vi "Auto-Generate-Docs.vi"(5 "Files Generated by Build":path[](array[path]), 6 "Top Level/Always Included VIs":path[](array[path]), 7 "Destination Path":path, 8 "error in (no error)":errorcluster, 9 "Target Name":string, 10 "Build Specification Name":string, 11 "Project Path":path) -> (0 "error out":errorcluster)   [LabVIEW 2019]
uses:
  <vilib>/printing/EasyPrintingControls.llb/custom_contents_options.ctl
  <vilib>/printing/EasyPrintingControls.llb/list_which_controls.ctl
  <vilib>/AppBuilder/AB_API_Simple/NI_App_Builder_API.lvlib
  <vilib>/AppBuilder/AB_API_Simple/Get Build Specification Version (path).vi
  <vilib>/Utility/NIReport.llb/NI_ReportGenerationCore.lvlib
panel:
  in  "custom contents options":T1={"include VI connector and icon"=TRUE, "include VI description"=TRUE, "include front panel"=FALSE, "surround front panel with border"=FALSE, "list of controls options"={"include list of controls"=FALSE, "list which controls?"=0, "include control descriptions?"=FALSE, "include control data types?"=FALSE}, "block diagram options"={"include block diagram"=FALSE, "hidden frames"=FALSE, "ordered (repeat from higher level if nested)"=FALSE}, "include VI hierarchy"=FALSE, "include list of subVIs"=FALSE, "include VI history"=FALSE, "include Express VI configuration information"=FALSE} {"list of controls options"."list which controls?" items=["all controls", "connected controls"]}
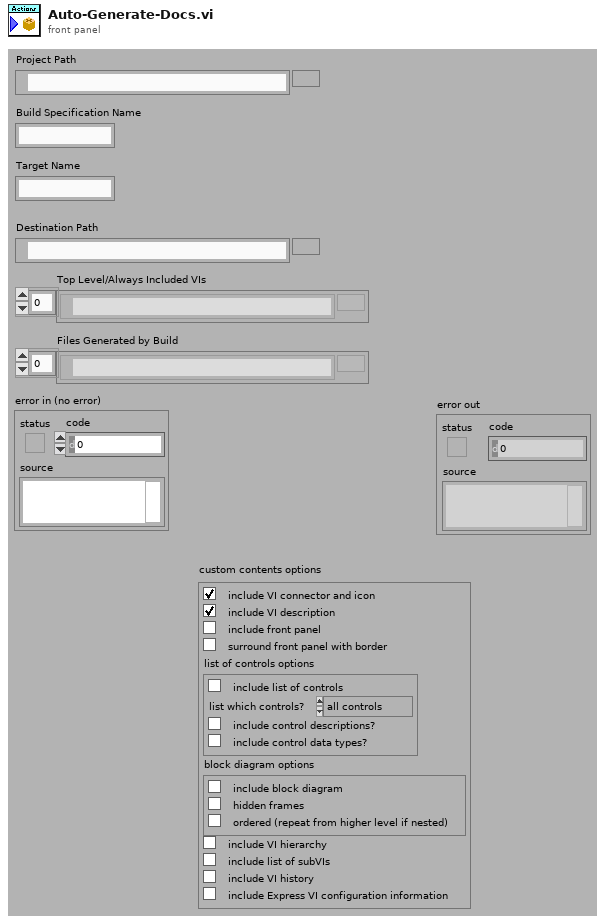
[diagram p1: front panel]
types:
  T1 = typedef "NI_ReportGenerationCore.lvlib/custom_contents_options.ctl" = cluster{"include VI connector and icon":bool, "include VI description":bool, "include front panel":bool, "surround front panel with border":bool, "list of controls options":cluster{"include list of controls":bool, "list which controls?":T2, "include control descriptions?":bool, "include control data types?":bool}, "block diagram options":cluster{"include block diagram":bool, "hidden frames":bool, "ordered (repeat from higher level if nested)":bool}, "include VI hierarchy":bool, "include list of subVIs":bool, "include VI history":bool, "include Express VI configuration information":bool}
  T2 = typedef "NI_ReportGenerationCore.lvlib/list_which_controls.ctl" = u16
  T3 = typedef "NI_App_Builder_API.lvlib/Build Specification Version.ctl" = cluster{"Major":u16, "Minor":u16, "Fix":u16, "Build":u16}
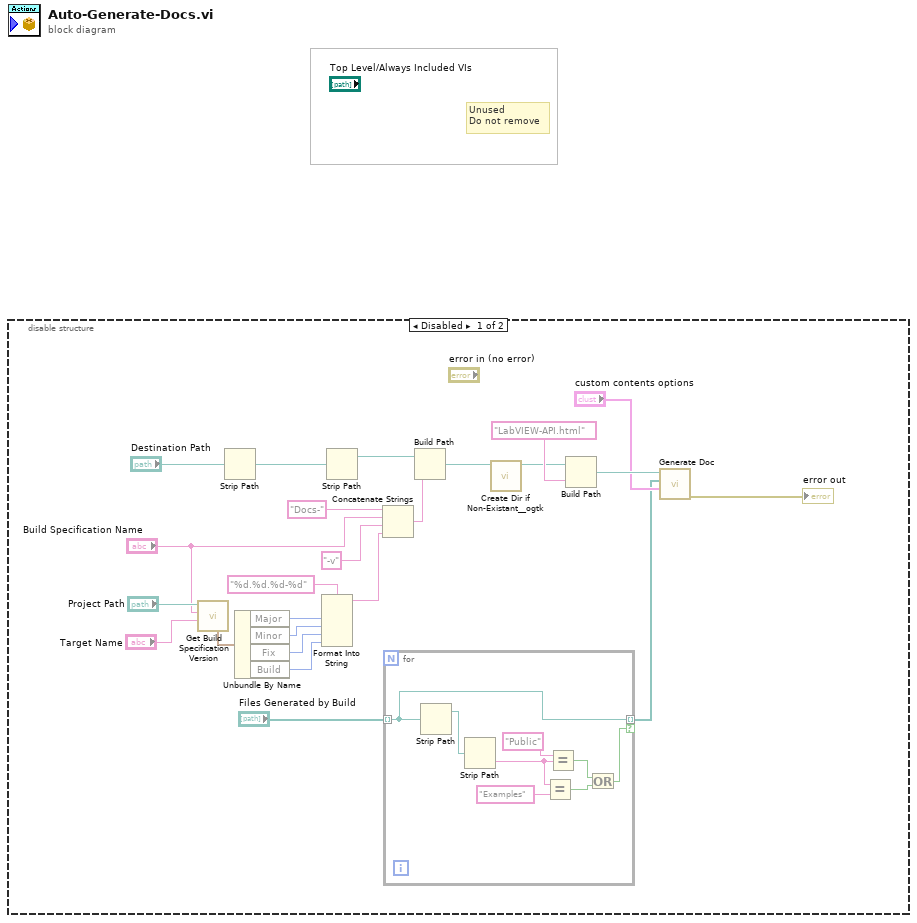
[diagram p0: block diagram]
diagram:
  # "Unused\nDo not remove"
  n1 = disable-structure shown="Disabled" {
    frame Disabled {
      n2 = call-poly <vilib>:"Get Build Specification Version.vi"("Name of target (My Computer)"="Target Name", "Name of build specification"="Build Specification Name", "Path to project"="Project Path") -> ("Build Specification Version"=w13:T3)  [unwired: 7 in, 1 out]
      n3 = Strip Path(path="Destination Path") -> (stripped path=w3:path)  [unwired: 1 out]
      n4 = Unbundle By Name(w13) -> ("Major"=w9:u16, "Minor"=w7:u16, "Fix"=w8:u16, "Build"=w6:u16)
      n5 = Format Into String(format string="%d.%d.%d-%d", w9, w7, w8, w6) -> (resulting string=w5:string)  [unwired: 2 in, 1 out]
      n6 = Strip Path(path=w3) -> (stripped path=w19:path)  [unwired: 1 out]
      n7 = Concatenate Strings("Docs-" ("name or relative path"), "Build Specification Name", "-v" ("name or relative path"), w5) -> (w15:string)
      n8 = for {
        tunnel: "Files Generated by Build" -> [w25] mode=indexing
        tunnel: [w25] -> w1 mode=indexing if=w26
        n9 = Strip Path(path=w25) -> (stripped path=w32:path)  [unwired: 1 out]
        n10 = Strip Path(path=w32) -> (name=w29:string)  [unwired: 1 out]
        n11 = Equal?(x=w29, y="Examples") -> (x = y?=w31:bool)
        n12 = Equal?(x="Public", y=w29) -> (x = y?=w30:bool)
        n13 = Or(x=w30, y=w31) -> (x .or. y?=w26:bool)
      }
      n14 = Build Path(base path=w19, name or relative path=w15) -> (appended path=w21:path)
      n15 = call <userlib>:"Create Dir if Non-Existant__ogtk.vi"("Directory Path"=w21) -> ("dup Directory Path"=w20:path)  [unwired: 8 in, 2 out]
      n16 = Build Path(base path=w20, name or relative path="LabVIEW-API.html") -> (appended path=w23:path)
      n17 = call "Generate Doc.vi"("custom contents options"="custom contents options", "Files Generated by Build"=w1, "appended path"=w23) -> ("error out"=→"error out":errorcluster)  [unwired: 8 in]
    }
    frame Enabled {
    }
  }
